vi "Graph Data.vi"(8 "error in (no error)":errorcluster, 10 "Leds 2":bool[](array[boolean]), 11 "Binary counter in":refnum<class "Binary counter.lvclass">) -> (0 "error out":errorcluster, 3 "Binary counter out":refnum<class "Binary counter.lvclass">)   [LabVIEW 2020, in "Binary counter.lvlib" / "Binary counter.lvclass"]
uses:
  Binary counter.lvclass
  Binary counter.lvclass/Binary counter.ctl
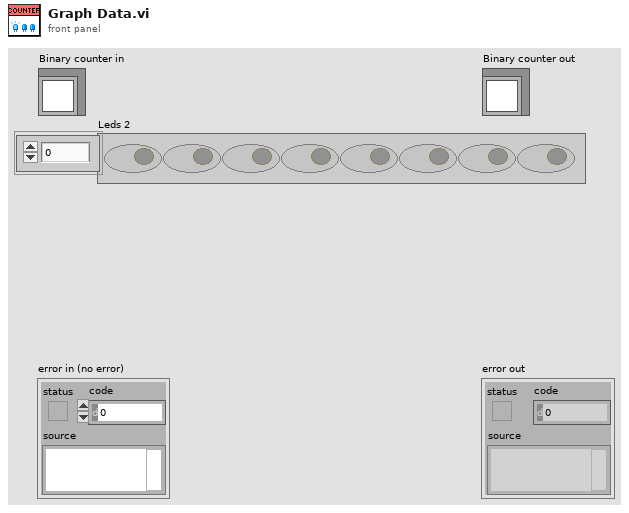
[diagram p1: front panel]
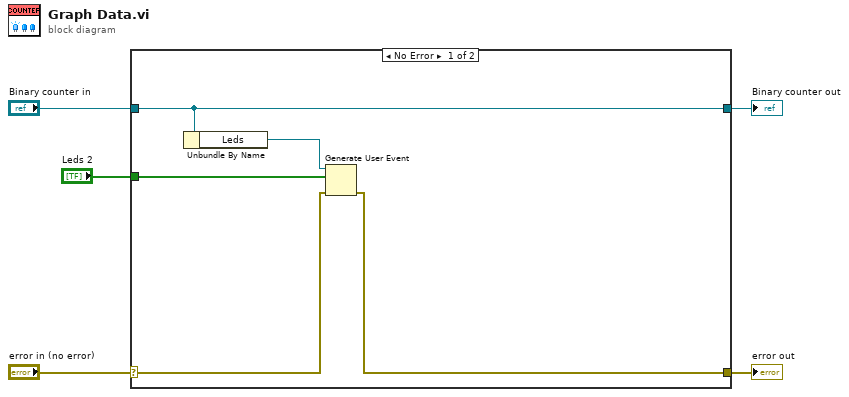
[diagram p0: block diagram]
diagram:
  n1 = case shown="No Error" "error in (no error)" {
    selector: "error in (no error)" -> [w7 w12]
    tunnel: [w6 w12] -> w4
    tunnel: [w10 w11] -> w2
    tunnel: "Binary counter in" -> [w10 w11]
    tunnel: "Leds 2" -> [w8 _]
    frame No Error {
      n2 = Unbundle By Name(w10) -> ("Leds"=w9:refnum<user-event>)
      n3 = Generate User Event(user event=w9, event data cluster=w8, error in=w7) -> (error out=w6:errorcluster)  [unwired: 1 in, 1 out]
    }
    frame Error {
    }
  }
  "error out" <- w4
  "Binary counter out" <- w2
